vi "Intake Logic.vi"() -> ()   [LabVIEW 2020]
uses:
  <vilib>/Rock Robotics/WPI/ThirdParty/Phoenix-LabVIEW/Motor Controller/Controls/CTRE_Phoenix_MotorControl_ControlMode.ctl
  <vilib>/Rock Robotics/WPI/ThirdParty/REV Robotics/REVLib/Typedef/Spark MAX Control Type.ctl
  <vilib>/Rock Robotics/WPI/Utilities/WPI_GetSetVariantRefNum.vi
  Robot Global Data.vi
  <vilib>/Rock Robotics/Network Tables/NT Read Numeric Array.vi
  2017 Swerve Code/Swerve Global Variables.vi
  <vilib>/addons/control/pid/pid.llb/PID (DBL).vi
  <vilib>/addons/control/pid/NI_PID_pid.lvlib
  <vilib>/ptbypt/NI_PtbyPt.lvlib
panel:
  in  "Enable Motor":bool
  in  "Angle Setpoint":dbl
  in  "output range":cluster{"output high":dbl, "output low":dbl}={"output high"=0.3, "output low"=-0.3} {"output low" format="%.2f"; "output high" format="%.2f"}
  in  "Shooter PID":T1={"P Gain"=0.0, "I Gain"=0.0, "D Gain"=0.0, "F Gain"=0.0, "I Zone"=0.0, "Min Output"=-1.0, "Max Output"=1.0}
  in  "Set PID":bool
  in  "Angle PID":T2={"proportional gain (Kc)"=0.04, "integral time (Ti, min)"=0.01, "derivative time (Td, min)"=0.0} {"derivative time (Td, min)" format="%.6f"; "integral time (Ti, min)" format="%.3f"; "proportional gain (Kc)" format="%.3f"}
  in  "speed lookup table":dbl[](array[numeric])
  out "Raspberry pi info":dbl[](array[numeric])
  in  "ball sense voltage":dbl=3.0 format="%#_13g"
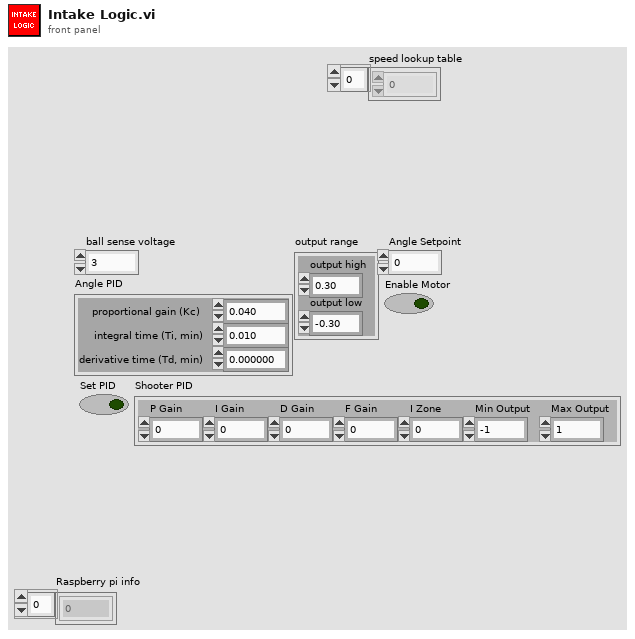
[diagram p1: front panel]
types:
  T1 = cluster{"P Gain":dbl, "I Gain":dbl, "D Gain":dbl, "F Gain":dbl, "I Zone":dbl, "Min Output":dbl, "Max Output":dbl}
  T2 = cluster{"proportional gain (Kc)":dbl, "integral time (Ti, min)":dbl, "derivative time (Td, min)":dbl}
  T3 = typedef "WPI_MotorControlDeviceRef.ctl" = cluster{"DeviceStatus":errorcluster, "Type":T4, "PWM":cluster{"PWM Channel":T5, "DeadBand":T6}, "CAN":cluster{"Device Number":u8, "SetOutput VI Ref":variant, "GetOutput VI Ref":variant, "Enable VI Ref":variant, "Disable VI Ref":variant, "Data":variant}, "Invert":bool, "DIO PWM":cluster{"PWM \"Enable\" Channel":T5, "DIOChannel":T7, "PWM Rate":dbl}}
  T4 = typedef "WPI_MotorControlType.ctl" = enum16{"PWM", "CAN", "DIO PWM"}
  T5 = typedef "FPGA_DIOPWMChannel.ctl" = enum8{"PWM 0", "PWM 1", "PWM 2", "PWM 3", "PWM 4", "PWM 5", "PWM 6", "PWM 7", "PWM 8", "PWM 9", "PWM MXP 0", "PWM MXP 1", "PWM MXP 2", "PWM MXP 3", "PWM MXP 4", "PWM MXP 5", "PWM MXP 6", "PWM MXP 7", "PWM MXP 8", "PWM MXP 9", "Invalid"}
  T6 = typedef "WPI_PWMDeadband.ctl" = cluster{"Name":string, "maxPositivePwm":i32, "minPositivePwm":i32, "centerPwm":i32, "maxNegativePwm":i32, "minNegativePwm":i32, "angularRange":u16}
  T7 = typedef "FPGA_DIOChannel.ctl" = enum8{"DIO 0", "DIO 1", "DIO 2", "DIO 3", "DIO 4", "DIO 5", "DIO 6", "DIO 7", "DIO 8", "DIO 9", "DIO MXP 0", "DIO MXP 1", "DIO MXP 2", "DIO MXP 3", "DIO MXP 4", "DIO MXP 5", "DIO MXP 6", "DIO MXP 7", "DIO MXP 8", "DIO MXP 9", "DIO MXP 10", "DIO MXP 11", "DIO MXP 12", "DIO MXP 13", "DIO MXP 14", "DIO MXP 15", "SPI Port CS1", "SPI Port CS2", "SPI Port CS3", "SPI Port MISO", "SPI Port MOSI", "Invalid"}
  T8 = typedef "WPI_AnalogChannelDevRef.ctl" = cluster{"DevStatus":errorcluster, "Analog Channel":T9}
  T9 = typedef "FPGA_AIChannel.ctl" = enum8{"AI 0", "AI 1", "AI 2", "AI 3", "AI MXP 0", "AI MXP 1", "AI MXP 2", "AI MXP 3", "Invalid"}
  T10 = typedef "Spark MAX Control Type.ctl" = enum16{"Percent VBus", "Voltage", "Velocity", "Position", "Smart Motion", "Current", "Smart Velocity"}
  T11 = typedef "CTRE_Phoenix_MotorControl_ControlMode.ctl" = u16
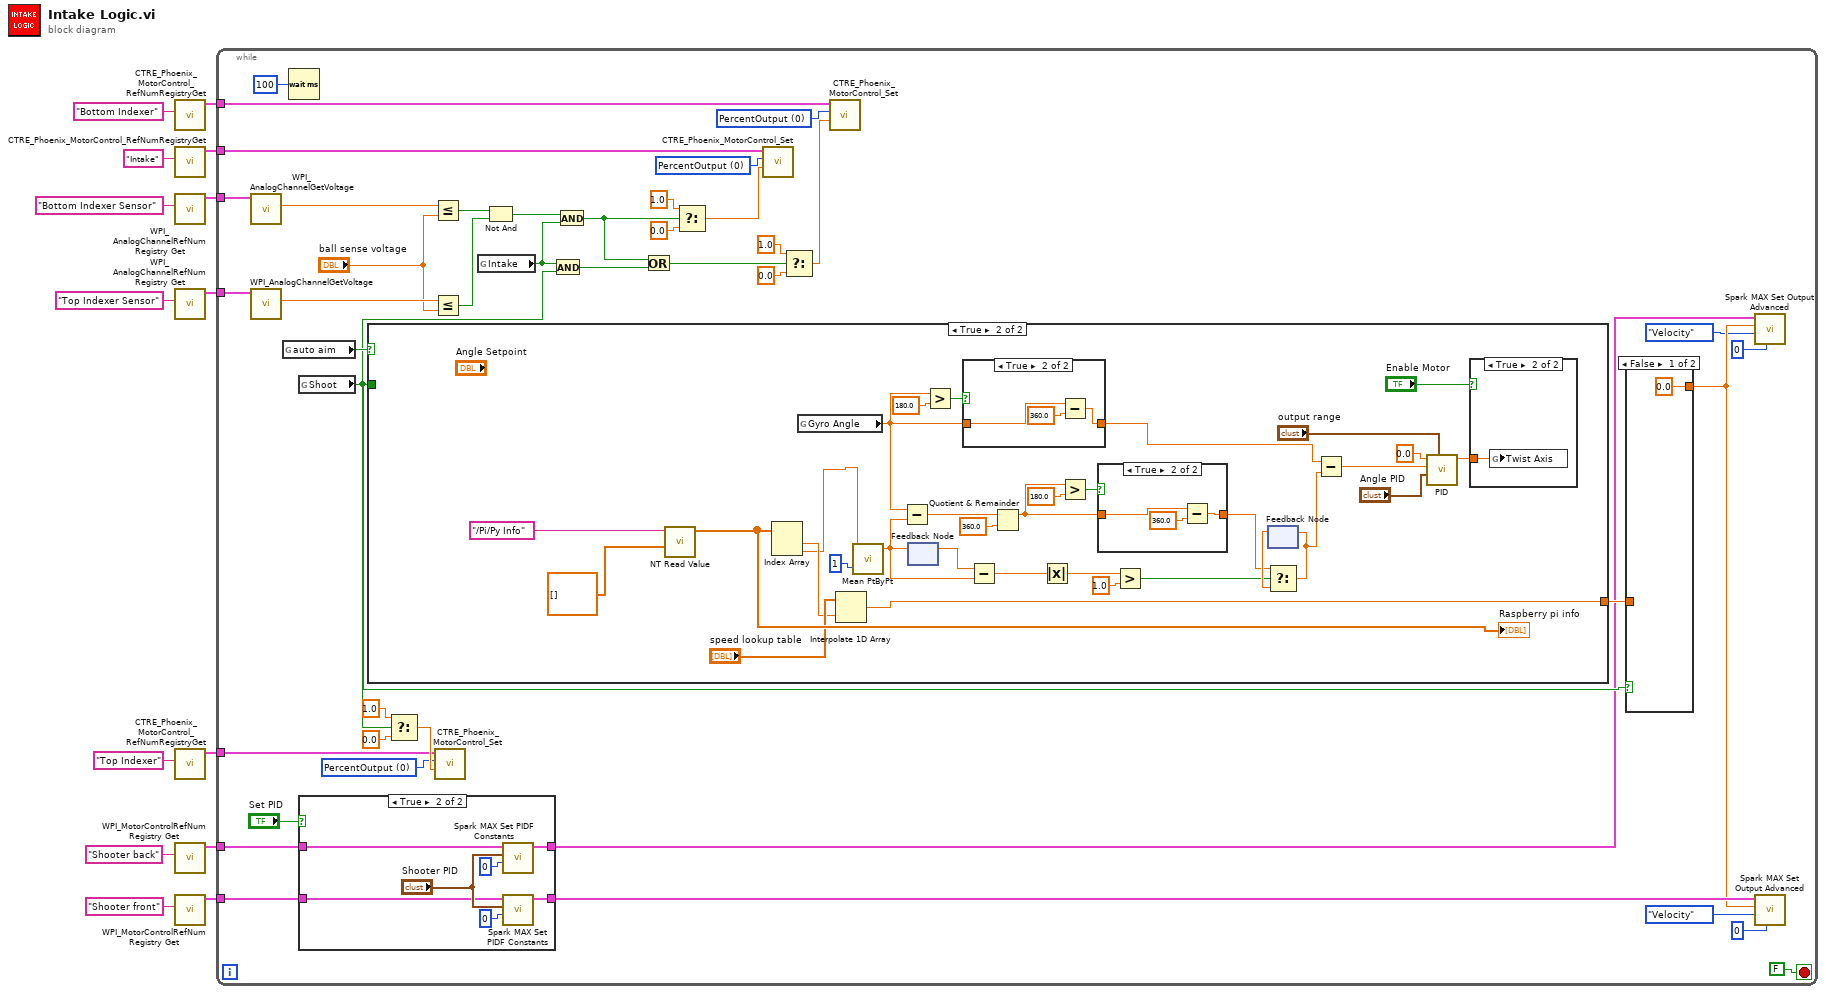
[diagram p0: block diagram]
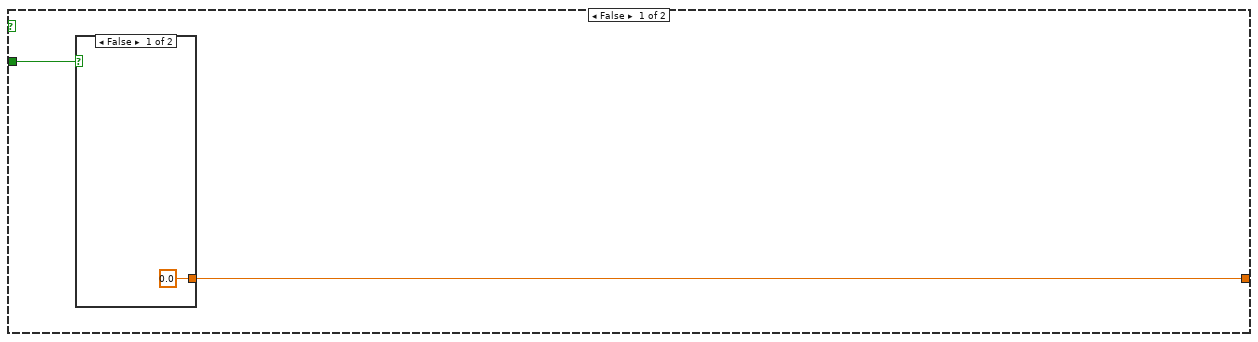
[diagram p4: hidden frame]
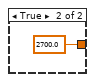
[diagram p5: hidden frame]
diagram:
  n1 = call <vilib>:"CTRE_Phoenix_MotorControl_RefNumRegistryGet.vi"("refnum name"="Bottom Indexer") -> ("PhoenixMotorControlDevRef"=w14:T3)  [unwired: 9 in, 1 out]
  n2 = call <vilib>:"CTRE_Phoenix_MotorControl_RefNumRegistryGet.vi"("refnum name"="Intake") -> ("PhoenixMotorControlDevRef"=w11:T3)  [unwired: 9 in, 1 out]
  n3 = call <vilib>:"WPI_AnalogChannelRefNum Registry Get.vi"("refnum name"="Bottom Indexer Sensor") -> ("AIDeviceRef"=w5:T8)  [unwired: 9 in, 1 out]
  n4 = call <vilib>:"WPI_AnalogChannelRefNum Registry Get.vi"("refnum name"="Top Indexer Sensor") -> ("AIDeviceRef"=w6:T8)  [unwired: 9 in, 1 out]
  n5 = call <vilib>:"CTRE_Phoenix_MotorControl_RefNumRegistryGet.vi"("refnum name"="Top Indexer") -> ("PhoenixMotorControlDevRef"=w9:T3)  [unwired: 9 in, 1 out]
  n6 = call <vilib>:"WPI_MotorControlRefNum Registry Get.vi"("refnum name"="Shooter back") -> ("MotorControlDevRef"=w2:T3)  [unwired: 9 in, 1 out]
  n7 = call <vilib>:"WPI_MotorControlRefNum Registry Get.vi"("refnum name"="Shooter front") -> ("MotorControlDevRef"=w1:T3)  [unwired: 9 in, 1 out]
  n8 = while {
    tunnel: w11 -> [w53]
    tunnel: w14 -> [w54]
    tunnel: w9 -> [w32]
    tunnel: w6 -> [w50]
    tunnel: w5 -> [w49]
    tunnel: w2 -> [w25]
    tunnel: w1 -> [w24]
    stop <- FALSE stop-if-true
    w31 = T11 0 items=["PercentOutput"=0, "Position"=1, "Velocity"=2, "Current"=3, "Follower"=5, "MotionProfile"=6, "MotionMagic"=7, "MotionProfileArc"=10, "Disabled"=15] ("Control Mode")
    w51 = T11 0 items=["PercentOutput"=0, "Position"=1, "Velocity"=2, "Current"=3, "Follower"=5, "MotionProfile"=6, "MotionMagic"=7, "MotionProfileArc"=10, "Disabled"=15] ("Control Mode")
    w52 = T11 0 items=["PercentOutput"=0, "Position"=1, "Velocity"=2, "Current"=3, "Follower"=5, "MotionProfile"=6, "MotionMagic"=7, "MotionProfileArc"=10, "Disabled"=15] ("Control Mode")
    n9 = call <vilib>:"WPI_AnalogChannelGetVoltage.vi"("AIDeviceRef"=w49) -> ("Voltage"=w48:dbl)  [unwired: 8 in, 2 out]
    n10 = call <vilib>:"WPI_AnalogChannelGetVoltage.vi"("AIDeviceRef"=w50) -> ("Voltage"=w47:dbl)  [unwired: 8 in, 2 out]
    n11 = global read "Robot Global Data.vi" "auto aim"() -> (w27:bool)
    n12 = Wait (ms)(milliseconds to wait=u32 100) -> ()  [unwired: 1 out]
    n13 = global read "Robot Global Data.vi" "Shoot"() -> (w22:bool)
    n14 = case shown="True" "Set PID" {
      tunnel: w25 -> [w60 w66]
      tunnel: w24 -> [w59 w65]
      tunnel: [w59 w62] -> w20
      tunnel: [w60 w61] -> w21
      frame False {
      }
      frame True {
        n15 = call <vilib>:"Spark MAX Set PIDF Constants.vi"("PIDF Slot"=0, "PID Constants"="Shooter PID", "MotorControlDeviceRef"=w66) -> ("MotorControlDeviceRef"=w61:T3)  [unwired: 7 in, 1 out]
        n16 = call <vilib>:"Spark MAX Set PIDF Constants.vi"("PIDF Slot"=0, "PID Constants"="Shooter PID", "MotorControlDeviceRef"=w65) -> ("MotorControlDeviceRef"=w62:T3)  [unwired: 7 in, 1 out]
      }
    }
    n17 = case shown="True" w27 {
      tunnel: [w68 w94] -> w23
      tunnel: w22 -> [w69 _]
      frame False {
        n18 = case shown="False" w69 {
          tunnel: [0.0 2700.0] -> w68
          frame False {
          }
          frame True {
          }
        }
      }
      frame True {
        n19 = call-poly <vilib>:"NT Read Value.vi"("Default Value"=dbl[] [], "Name"="/Pi/Py Info") -> ("Numeric Array"=w101:dbl[])  [unwired: 8 in, 1 out]
        "Raspberry pi info" <- w101
        n20 = Index Array(array=w101) -> (element #1=w99:dbl, element #2=w72:dbl)  [unwired: 2 in]
        n21 = global read "Swerve Global Variables.vi" "Gyro Angle"() -> (w86:dbl)
        n22 = Interpolate 1D Array(1:w99, 2:"speed lookup table") -> (0:w94:dbl)
        n23 = call <vilib>:"Mean PtByPt.vi"("x"=w72, "sample length"=1) -> ("mean"=w79:dbl)  [unwired: 2 in, 1 out]
        n24 = Subtract(x=w86, y=w79) -> (x-y=w85:dbl)
        n25 = feedback-in #1(w79) -> ()
        n26 = feedback #1() -> (w88:dbl)  [unwired: 1 in]
        n27 = Greater?(x=w86, y=180.0) -> (0:w92:bool)
        n28 = case shown="True" w92 {
          tunnel: w86 -> [w109 w111]
          tunnel: [w109 w110] -> w91
          frame False {
          }
          frame True {
            n29 = Subtract(x=w111, y=360.0) -> (x-y=w110:dbl)
          }
        }
        n30 = Subtract(x=w88, y=w79) -> (x-y=w78:dbl)
        n31 = Quotient & Remainder(x=w85, y=360.0) -> (x-y*floor(x/y)=w81:dbl)  [unwired: 1 out]
        n32 = Absolute Value(x=w78) -> (abs(x)=w77:dbl)
        n33 = Greater?(x=w81, y=180.0) -> (0:w82:bool)
        n34 = case shown="True" w82 {
          tunnel: [w104 w105] -> w74
          tunnel: w81 -> [w104 w107]
          frame False {
          }
          frame True {
            n35 = Subtract(x=w107, y=360.0) -> (x-y=w105:dbl)
          }
        }
        n36 = Greater?(x=w77, y=1.0) -> (0:w75:bool)
        n37 = feedback #2() -> (w87:dbl)  [unwired: 1 in]
        n38 = Select(t=w74, s=w75, f=w87) -> (s? t:f=w73:dbl)
        n39 = feedback-in #2(w73) -> ()
        n40 = Subtract(x=w91, y=w73) -> (x-y=w96:dbl)
        n41 = call-poly <vilib>:"PID.vi"("output range"="output range", "PID gains"="Angle PID", "process variable"=w96, "setpoint"=0.0) -> ("output"=w95:dbl)  [unwired: 6 in, 1 out]
        n42 = case shown="True" "Enable Motor" {
          tunnel: w95 -> [_ w108]
          frame False {
          }
          frame True {
            n43 = global write "Swerve Global Variables.vi" "Twist Axis"(w108) -> ()
          }
        }
      }
    }
    n44 = Select(t=1.0, s=w22, f=0.0) -> (s? t:f=w33:dbl)
    n45 = Less Or Equal?(x=w48, y="ball sense voltage") -> (x <= y?=w44:bool)
    n46 = Less Or Equal?(x=w47, y="ball sense voltage") -> (x <= y?=w45:bool)
    n47 = call <vilib>:"CTRE_Phoenix_MotorControl_Set.vi"("Output"=w33, "Control Mode"=w31, "PhoenixMotorControlDevRef"=w32) -> ()  [unwired: 7 in, 2 out]
    n48 = global read "Robot Global Data.vi" "Intake"() -> (w29:bool)
    n49 = Not And(1:w45, 2:w44) -> (0:w28:bool)
    n50 = And(x=w29, y=w22) -> (x .and. y?=w37:bool)
    n51 = And(x=w28, y=w29) -> (x .and. y?=w30:bool)
    n52 = Or(x=w30, y=w37) -> (x .or. y?=w36:bool)
    n53 = Select(t=1.0, s=w30, f=0.0) -> (s? t:f=w35:dbl)
    n54 = call <vilib>:"CTRE_Phoenix_MotorControl_Set.vi"("Output"=w35, "Control Mode"=w52, "PhoenixMotorControlDevRef"=w53) -> ()  [unwired: 7 in, 2 out]
    n55 = Select(t=1.0, s=w36, f=0.0) -> (s? t:f=w34:dbl)
    n56 = call <vilib>:"CTRE_Phoenix_MotorControl_Set.vi"("Output"=w34, "Control Mode"=w51, "PhoenixMotorControlDevRef"=w54) -> ()  [unwired: 7 in, 2 out]
    n57 = case shown="False" w22 {
      tunnel: [0.0 w58] -> w19
      tunnel: w23 -> [_ w58]
      frame False {
      }
      frame True {
      }
    }
    n58 = call <vilib>:"Spark MAX Set Output Advanced.vi"("PIDF Slot (0)"=0, "Control Mode"=Spark_MAX_Control_Type."Velocity", "Setpoint"=w19, "MotorControlDevRef"=w21) -> ()  [unwired: 6 in, 2 out]
    n59 = call <vilib>:"Spark MAX Set Output Advanced.vi"("PIDF Slot (0)"=0, "Control Mode"=Spark_MAX_Control_Type."Velocity", "Setpoint"=w19, "MotorControlDevRef"=w20) -> ()  [unwired: 6 in, 2 out]
  }
